vi "write_buffer_to_file.vi"(8 "error in (no error)":errorcluster, 10 "data_logger.lvclass":refnum<class "data_logger.lvclass">, 11 "picoharp in":refnum<class "picoharp.lvclass">) -> (0 "error out":errorcluster, 1 "Stream_done":bool, 2 "data_logger.lvclass 2":refnum<class "data_logger.lvclass">, 3 "picoharp out":refnum<class "picoharp.lvclass">)   [LabVIEW 2015, in "picoharp.lvclass"]
uses:
  picoharp.lvclass
  Data Logger Class/data_logger.lvclass
  picoharp.lvclass/picoharp.ctl
  lvoop_dll-master/picoquant_Tmodes.ctl
  lvoop_dll-master/picoquant_devices.ctl
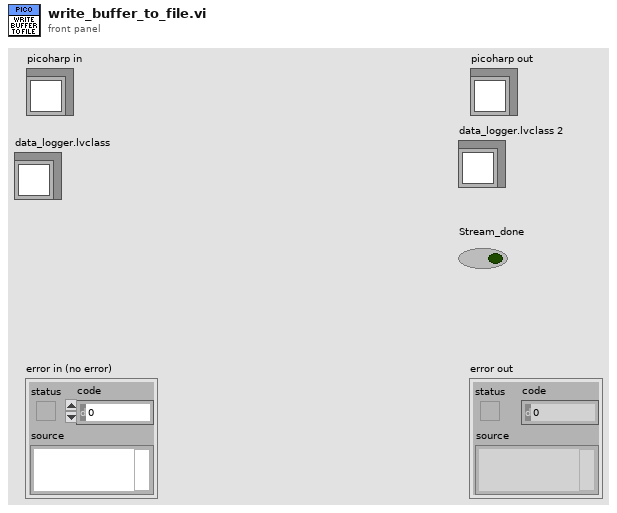
[diagram p1: front panel]
types:
  T1 = typedef "picoquant_devices.ctl" = enum16{"hydraharp", "picoharp"}
  T2 = typedef "hpanel_acq_modes.ctl" = u16
  T3 = typedef "picoquant_Tmodes.ctl" = u16
  T4 = typedef "hydraharp_fifo_queue_data.ctl" = cluster{"fifo_buffer":u32[], "fifo_action":T5}
  T5 = typedef "hydraharp_fifo_actions.ctl" = enum16{"stop", "new_data"}
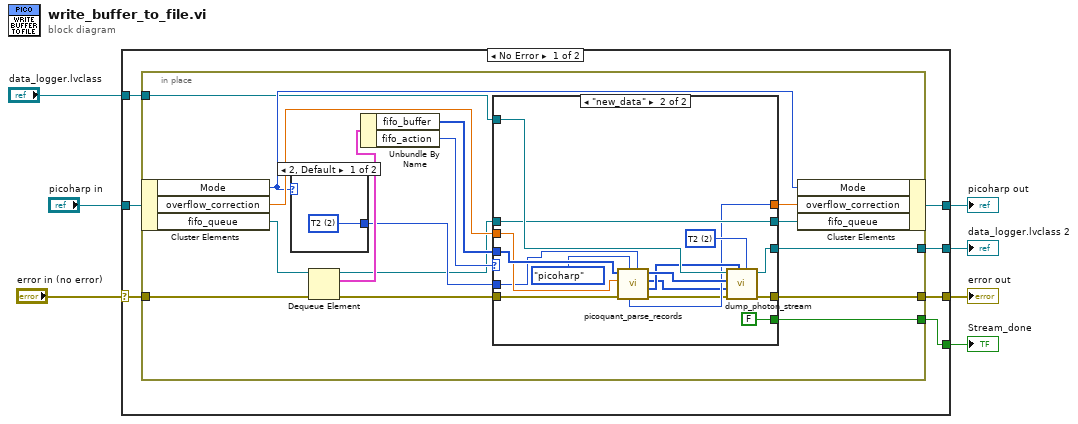
[diagram p0: block diagram]
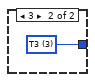
[diagram p2: hidden frame]
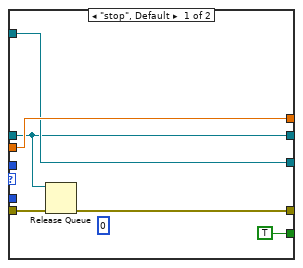
[diagram p3: hidden frame]
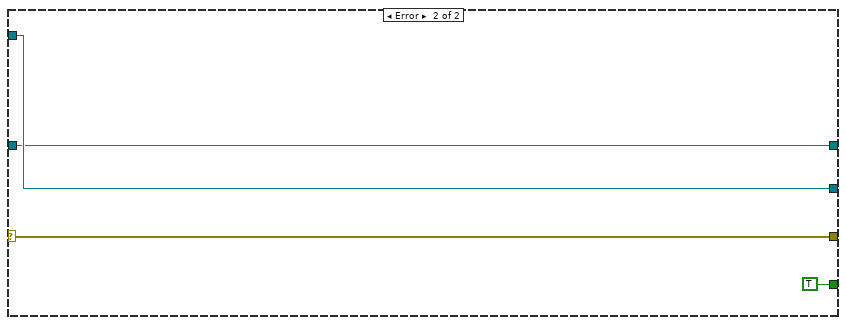
[diagram p4: hidden frame]
diagram:
  n1 = case shown="No Error" "error in (no error)" {
    selector: "error in (no error)" -> [w13 w55]
    tunnel: "data_logger.lvclass" -> [w10 w58]
    tunnel: "picoharp in" -> [w14 w57]
    tunnel: [w12 w57] -> w4
    tunnel: [w9 w58] -> w2
    tunnel: [w11 TRUE] -> w3
    tunnel: [w8 w55] -> w1
    frame No Error {
      n2 = in-place {
        in-place-border: w13 -> [w29]
        in-place-border: [w20] -> w11
        in-place-border: [w19] -> w8
        in-place-border: w10 -> [w18]
        in-place-border: [w17] -> w9
        n3 = in-place-cluster #1(w14) -> ("Mode"=w21:T2, "overflow_correction"=w25:dbl, "fifo_queue"=w30:refnum<queue>)
        n4 = case shown="2, Default" w21 {
          tunnel: [w31 w32] -> w23
          frame 2, Default {
            w31 = T3 2 items=["T2"=2, "T3"=3] ("acq_mode")
          }
          frame 3 {
            w32 = T3 3 items=["T2"=2, "T3"=3] ("acq_mode")
          }
        }
        n5 = Dequeue Element(queue=w30, error in (no error)=w29) -> (queue out=w16:refnum<queue>, element=w28:T4, error out=w24:errorcluster)  [unwired: 1 in, 1 out]
        n6 = Unbundle By Name(w28) -> ("fifo_buffer"=w26:u32[], "fifo_action"=w27:T5)
        n7 = case shown="\"new_data\"" w27 {
          tunnel: w26 -> [_ w46]
          tunnel: w25 -> [w38 w45]
          tunnel: w24 -> [w35 w48]
          tunnel: w23 -> [_ w42]
          tunnel: [w38 w41] -> w22
          tunnel: [TRUE FALSE] -> w20
          tunnel: [w34 w53] -> w19
          tunnel: w18 -> [w36 w52]
          tunnel: [w36 w51] -> w17
          tunnel: w16 -> [w33 w50]
          tunnel: [w33 w50] -> w15
          frame "stop", Default {
            (unwired) u64 0 ("photon_count")
            n8 = Release Queue(queue=w33, error in (no error)=w35) -> (error out=w34:errorcluster)  [unwired: 1 in, 2 out]
          }
          frame "new_data" {
            w49 = T3 2 items=["T2"=2, "T3"=3] ("acq_mode")
            n9 = call "picoquant_parse_records.vi"("acq_mode"=w42, "Device"=picoquant_devices."picoharp", "error in (no error)"=w48, "overflow"=w45, "fifo_buffer"=w46) -> ("error out"=w40:errorcluster, "sync"=w43:u64[], "channels"=w39:u8[], "times"=w47:u64[], "overflow"=w41:u64)  [unwired: 1 in, 1 out]
            n10 = call-dynamic "dump_photon_stream.vi"("Ring"=w49, "sync"=w43, "error in (no error)"=w40, "channels"=w39, "photon_records"=w47, "data_logger in"=w52) -> ("error out"=w53:errorcluster, "data_logger out"=w51:refnum<class "data_logger.lvclass">)  [unwired: 4 in]
          }
        }
        n11 = in-place-cluster #1("Mode"=w21, "overflow_correction"=w22, "fifo_queue"=w15) -> (w12:refnum<class "picoharp.lvclass">)
      }
    }
    frame Error {
    }
  }
  "error out" <- w1
  "picoharp out" <- w4
  "data_logger.lvclass 2" <- w2
  "Stream_done" <- w3
